vi "Ping.vi"(1 "PC Name or IP Address":string) -> (0 "Available":bool)   [LabVIEW 2013]
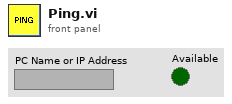
[diagram p1: front panel]
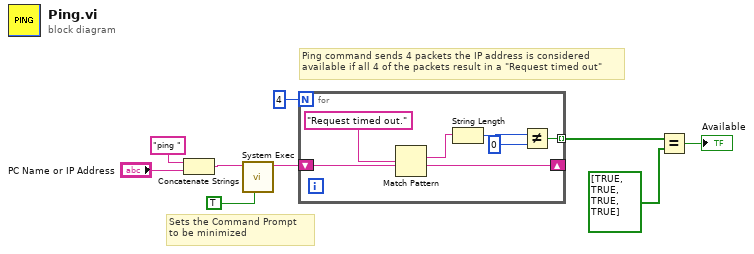
[diagram p0: block diagram]
diagram:
  # "Sets the Command Prompt\nto be minimized"
  # "Ping command sends 4 packets the IP address is considered\navailable if all 4 of the packets result in a \"Request timed out\""
  n1 = Concatenate Strings("ping " ("command line"), "PC Name or IP Address") -> (w3:string)
  n2 = call <vilib>:"System Exec.vi"("run minimized? (F)"=TRUE, "command line"=w3) -> ("standard output"=w2:string)  [unwired: 6 in, 3 out]
  n3 = for {
    N: 4 -> [_]
    shift-right: [w14] -> _
    shift-left: w2 -> [w15]
    tunnel: [w10] -> w6 mode=indexing
    n4 = Match Pattern(string=w15, regular expression="Request timed out.") -> (match substring=w13:string, after substring=w14:string)  [unwired: 1 in, 2 out]
    n5 = String Length(string=w13) -> (length=w12:i32)
    n6 = Not Equal?(x=w12, y=0) -> (x != y?=w10:bool)
  }
  n7 = Equal?(x=w6, y=bool[] [TRUE, TRUE, TRUE, TRUE]) -> (x = y?=→"Available":bool)
